vi "Get Tx Generic Payload Entry List.vi"(8 "error in":errorcluster, 11 "custom device ref in":T3 format="%.0x") -> (0 "error out":errorcluster, 2 "Payload Entry List":T1[](array[typedef]) {"Parameters"."encoding" items=["BNR", "BCD", "Discrete"]}, 3 "custom device ref out":T3 format="%.0x", 4 "Found?":bool)   [LabVIEW 2020, in "AIM ARINC 664 Scripting.lvlib"]
uses:
  AIM ARINC 664 Scripting.lvlib
  Constants.vi
  <vilib>/NI VeriStand/Custom Device Tools/Custom Device Utility Library/Custom Device Utility Library.lvlib
  <vilib>/NI VeriStand/Custom Device API/Custom Device API.lvlib
  Shared/Frame Payload Parameters.ctl
  <vilib>/NI VeriStand/Custom Device API/Get Item Property (U32 Array).vi
  <vilib>/NI VeriStand/Custom Device Tools/Custom Device Utility Library/NI VeriStand - Search for Item by GUID.vi
  <vilib>/NI VeriStand/Custom Device Tools/Custom Device Utility Library/NI VeriStand - Search for All Items by GUID.vi
  <vilib>/NI VeriStand/Custom Device API/Get Item Property (String).vi
  Shared/Encoding (Arinc664).ctl
  <vilib>/NI VeriStand/Custom Device API/Custom Device Item Ref.ctl
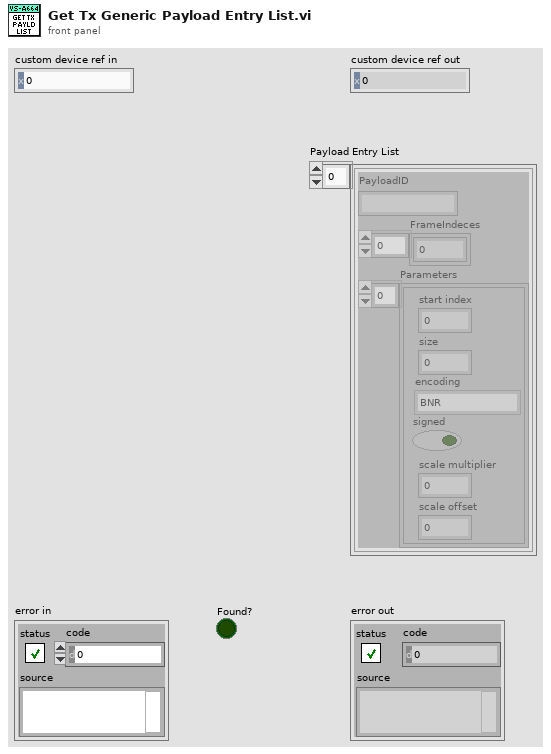
[diagram p1: front panel]
types:
  T1 = typedef "Frame Payload Parameters.ctl" = cluster{"PayloadID":string, "FrameIndeces":u32[], "Parameters":cluster{"start index":i32, "size":i32, "encoding":T2, "signed":bool, "scale multiplier":dbl, "scale offset":dbl}[]}
  T2 = typedef "Encoding (Arinc664).ctl" = u16
  T3 = typedef "Custom Device API.lvlib/Custom Device Item Ref.ctl" = u64
  T4 = cluster{"start index":i32, "size":i32, "encoding":T2, "signed":bool, "scale multiplier":dbl, "scale offset":dbl}
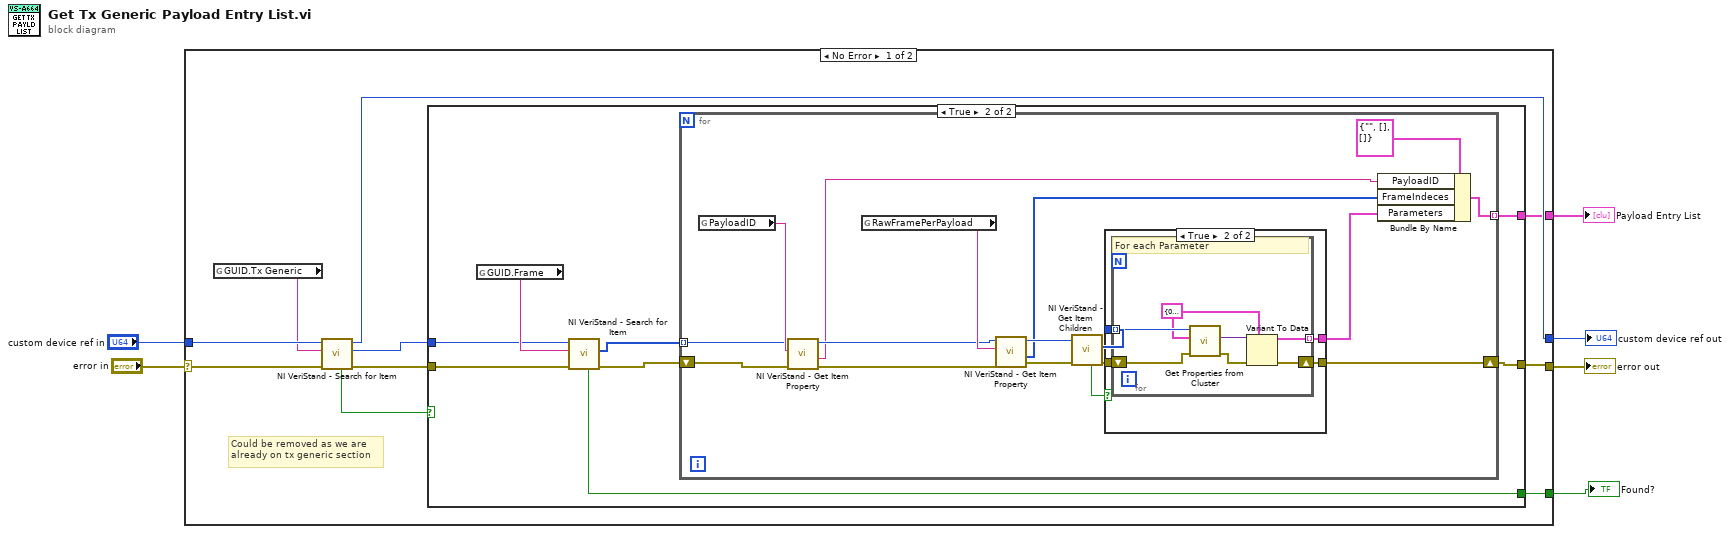
[diagram p0: block diagram]
diagram:
  n1 = case shown="No Error" "error in" {
    selector: "error in" -> [w15 w56]
    tunnel: "custom device ref in" -> [w16 w55]
    tunnel: [w9 w56] -> w5
    tunnel: [w13 w55] -> w4
    tunnel: [w8 _] -> w2
    tunnel: [w7 _] -> w1
    frame No Error {
      # "Could be removed as we are\nalready on tx generic section"
      n2 = global read "Constants.vi" "GUID.Tx Generic"() -> (w14:string)
      n3 = call-poly <vilib>:"NI VeriStand - Search for Item.vi"("error in"=w15, "Item GUID"=w14, "Section Ref in"=w16) -> ("error out"=w12:errorcluster, "Item Ref"=w11:T3, "Section Ref out"=w13:T3, "Found"=w10:bool)  [unwired: 5 in]
      n4 = case shown="True" w10 {
        tunnel: w12 -> [w17 w20]
        tunnel: w11 -> [_ w19]
        tunnel: [w17 w22] -> w9
        tunnel: [_ w21] -> w8
        tunnel: [_ w18] -> w7
        frame False {
        }
        frame True {
          n5 = global read "Constants.vi" "GUID.Frame"() -> (w25:string)
          n6 = call-poly <vilib>:"NI VeriStand - Search for Item.vi"("error in"=w20, "Item GUID"=w25, "Section Ref in"=w19) -> ("error out"=w24:errorcluster, "Item Refs"=w23:T3[], "Found"=w18:bool)  [unwired: 5 in, 1 out]
          n7 = for {
            tunnel: w23 -> [w30] mode=indexing
            shift-right: [w36] -> w22
            shift-left: w24 -> [w31]
            tunnel: [w33] -> w21 mode=indexing
            n8 = global read "Constants.vi" "PayloadID"() -> (w32:string)
            n9 = call-poly <vilib>:"NI VeriStand - Get Item Property.vi"("error in (no error)"=w31, "Property Name"=w32, "Item Ref in"=w30) -> ("error out"=w29:errorcluster, "Value"=w27:string, "Item Ref out"=w28:T3)  [unwired: 5 in, 1 out]
            n10 = global read "Constants.vi" "RawFramePerPayload"() -> (w42:string)
            n11 = call-poly <vilib>:"NI VeriStand - Get Item Property.vi"("error in (no error)"=w29, "Property Name"=w42, "Item Ref in"=w28) -> ("error out"=w38:errorcluster, "Value"=w26:u32[], "Item Ref out"=w39:T3)  [unwired: 5 in, 1 out]
            n12 = call <vilib>:"NI VeriStand - Get Item Children.vi"("error in (no error)"=w38, "Item Ref in"=w39) -> ("error out"=w41:errorcluster, "Child Refs"=w40:T3[], "Found"=w37:bool)  [unwired: 6 in, 1 out]
            n13 = case shown="True" w37 {
              tunnel: w41 -> [w43 w47]
              tunnel: w40 -> [_ w46]
              tunnel: [w43 w45] -> w36
              tunnel: [_ w44] -> w34
              frame False {
              }
              frame True {
                n14 = for {
                  tunnel: w46 -> [w52] mode=indexing
                  shift-right: [w49] -> w45
                  shift-left: w47 -> [w50]
                  tunnel: [w51] -> w44 mode=indexing
                  w48 = T4 {"start index"=0, "size"=0, "encoding"=0, "signed"=FALSE, "scale multiplier"=0.0, "scale offset"=0.0} ("Parameter")
                  # "For each Parameter"
                  n15 = call "Get Properties from Cluster.vi"("error in"=w50, "Variant Cluster"=w48, "custom device ref in"=w52) -> ("error out"=w53:errorcluster, "data"=w54:variant)  [unwired: 5 in, 2 out]
                  n16 = Variant To Data(error in=w53, type=w48, Variant=w54) -> (data=w51:T4, error out=w49:errorcluster)
                }
              }
            }
            n17 = Bundle By Name(cluster=T1 {"PayloadID"="", "FrameIndeces"=[], "Parameters"=[]} ("Cluster"), "PayloadID"=w27, "FrameIndeces"=w26, "Parameters"=w34) -> (w33:T1)
          }
        }
      }
    }
    frame Error {
    }
  }
  "error out" <- w5
  "custom device ref out" <- w4
  "Found?" <- w1
  "Payload Entry List" <- w2
